vi "Gaussmeter425_BvsTime_HeliumEdition.vi"() -> ()   [LabVIEW 2014]
uses:
  <vilib>/Platform/TimedLoop/XDataNode/timing_clust.ctl
  <vilib>/Platform/TimedLoop/XDataNode/nitl_modes.ctl
  <vilib>/Platform/TimedLoop/XDataNode/wakeup.ctl
  <instrlib>/Agilent 3446X Series/Public/Data/Read (Single Point).vi
  <instrlib>/Lake Shore 425/Public/Data/Field Data (Single Reading).vi
  <vilib>/Utility/file.llb/Write To Spreadsheet File (DBL).vi
  <vilib>/Platform/TimedLoop/XDataNode/XDataNode.xnode
  <instrlib>/Lake Shore 425/Lake Shore 425.lvlib
  <vilib>/Platform/TimedLoop/XDataNode/XDNodeRunTimeDep.lvlib
  <instrlib>/Agilent 3446X Series/Agilent 3446X Series.lvlib
panel:
  out "Output file name":string
  in  "Use multimeter ON / OFF":bool=TRUE
  in  "Comments":string
  in  "Setup":string(combo)
  out "?":dbl(graph)
  in  "VISA resource name MM":refnum<visa-resource-name>="USB0::0x0957::0x1A07::MY53203201::INSTR"
  in  "Measurement Function (10: Voltage DC)":i32(ring)=10 items=["Continuity", "Current AC", "Current DC", "Diode", "Frequency", "Resistance 4-wire", "Period", "Resistance 2-wire", "Temperature", "Voltage AC", "Voltage DC", "Voltage DC Ratio"]
  out "Current [A]":dbl
  out "Magnetic Flux [mT]":dbl
  in  "day":dbl
  in  "h":dbl
  in  "min":dbl
  in  "sec":dbl
  out "Time since run start [s]":dbl
  in  "VISA resource name GM":refnum<visa-resource-name>="COM4"
  in  "Measurements per second:":dbl=1.0
  out "?":dbl(graph)
  in  "?":bool
  in  "Serial Configuration":T1={"Baud Rate"=57600, "Parity"=1, "Data Bits"=7, "Stop Bits"=10, "Flow Control"=0} {"Flow Control" items=["None", "XON/XOFF", "RTS/CTS", "XON/XOFF & RTS/CTS", "DTR/DSR", "XON/XOFF & DTR/DSR"]; "Stop Bits" items=["1.0"=10, "1.5"=15, "2.0"=20]; "Data Bits" items=["7"=7, "8"=8]; "Parity" items=["None", "Odd", "Even", "Mark", "Space"]; "Baud Rate" items=["300"=300, "600"=600, "1200"=1200, "2400"=2400, "4800"=4800, "9600"=9600, "19200"=19200, "38400"=38400, "57600"=57600]}
  # "Automatically stop after..."
  # "more than 3 may not work"
  # "Gaussmeter"
  # "Multimeter"
  # "USB0::0x0957: for multimeter"
  # "Voltage DC for Amp"
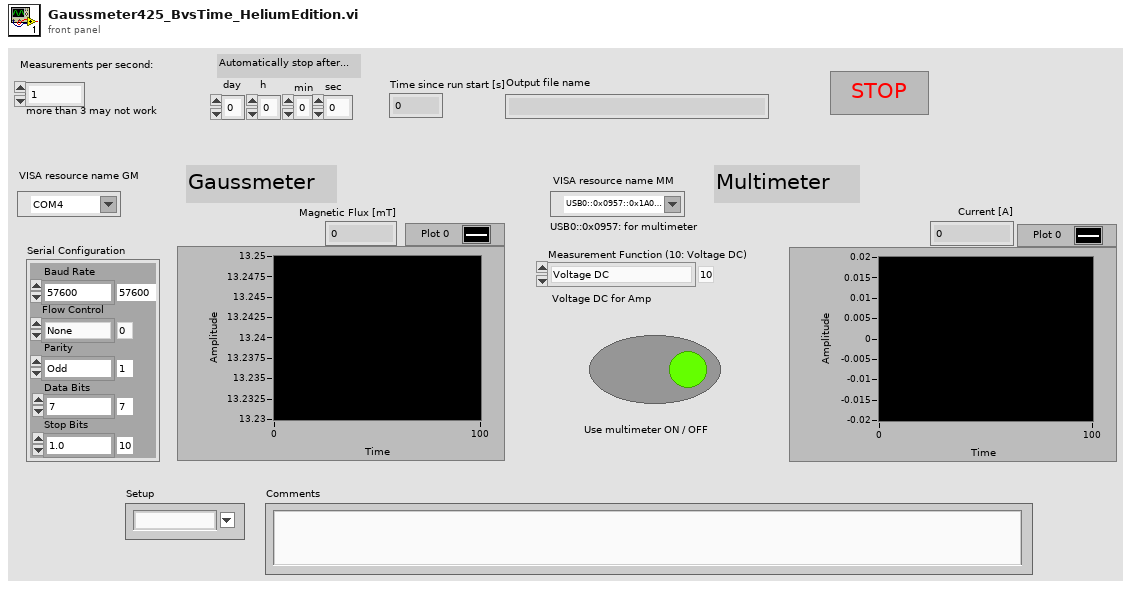
[diagram p1: front panel]
types:
  T1 = cluster{"Baud Rate":u32, "Parity":u16, "Data Bits":u16, "Stop Bits":u16, "Flow Control":u16}
  T2 = typedef "XDNodeRunTimeDep.lvlib/timing_clust.ctl" = cluster{"Expected End [f-1]":u64, "Actual End [f-1]":u64, "Finished Late? [f-1]":bool, "Expected End [i-1]":u64, "Actual End [i-1]":u64, "Finished Late? [i-1]":bool, "Expected Start [i]":u64, "Actual Start [i]":u64, "Expected Start [f]":u64, "Actual Start [f]":u64, "Source Name":string, "Structure Name":string, "Period":i64, "Deadline":i64, "Offset":i64, "Start":i64, "Priority":i32, "Timeout":i32, "Mode":T3, "Wakeup Reason":T4, "Error":errorcluster, "Source Type":string, "Secondary Source Type":string, "Global End Time":u64, "Global Start Time":u64, "Frame Duration":u64, "Iteration Duration":u64, "Assigned CPU":i32, "I/O Scan Engine Mode":u32}
  T3 = typedef "XDNodeRunTimeDep.lvlib/nitl_modes.ctl" = enum32{"No Change", "Process missed periods, maintain original phase", "Discard missed periods, maintain original phase", "Process missed periods, ignore original phase", "Discard missed periods, ignore original phase"}
  T4 = typedef "XDNodeRunTimeDep.lvlib/wakeup.ctl" = enum32{"Normal", "Aborted", "Asynchronous wakeup", "Timing source error", "Timed loop error", "Timeout"}
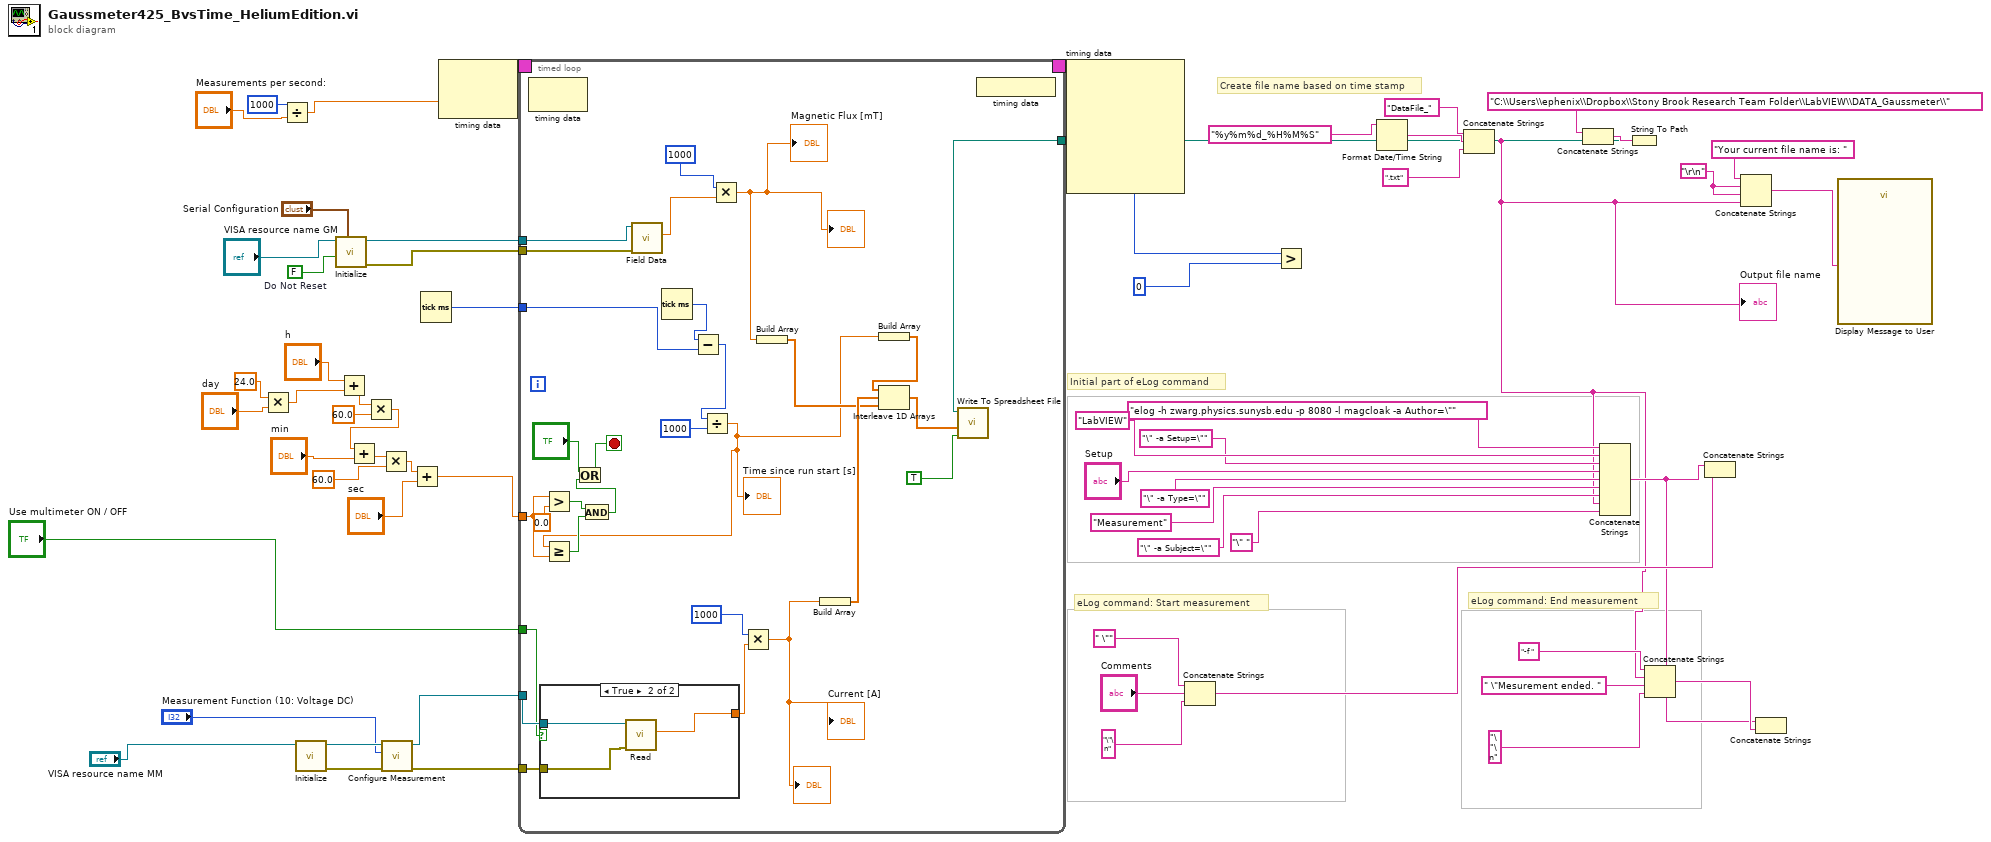
[diagram p0: block diagram]
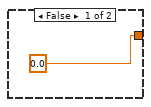
[diagram p2: hidden frame]
diagram:
  w46 = "\r\n"
  w60 = FALSE  # Do Not Reset
  # "eLog command: End measurement"
  # "eLog command: Start measurement"
  # "Initial part of eLog command"
  # "Create file name based on time stamp"
  n1 = Multiply(x=24.0, y="day") -> (x*y=w41:dbl)
  n2 = Divide(x=1000, y="Measurements per second:") -> (x/y=w44:dbl)
  n3 = call <instrlib>:"Initialize.vi"("VISA resource name"="VISA resource name MM") -> ("error out"=w30:errorcluster, "VISA resource name out"=w31:refnum<visa-resource-name>)  [unwired: 4 in, 5 out]
  n4 = call <instrlib>:"Initialize.vi"("Serial Configuration"="Serial Configuration", "Reset (True)"=w60, "VISA resource name"="VISA resource name GM") -> ("error out"=w57:errorcluster, "VISA resource name out"=w58:refnum<visa-resource-name>)  [unwired: 7 in]
  n5 = Add(x="h", y=w41) -> (x+y=w40:dbl)
  n6 = Multiply(x=w40, y=60.0) -> (x*y=w38:dbl)
  n7 = Add(x=w38, y="min") -> (x+y=w36:dbl)
  n8 = Multiply(x=w36, y=60.0) -> (x*y=w34:dbl)
  n9 = call <instrlib>:"Configure Measurement.vi"("error in (no error)"=w30, "Measurement Function (10: Voltage DC)"="Measurement Function (10: Voltage DC)", "VISA resource name"=w31) -> ("error out"=w26:errorcluster, "VISA resource name out"=w27:refnum<visa-resource-name>)  [unwired: 3 in, 4 out]
  n10 = Add(x=w34, y="sec") -> (x+y=w32:dbl)
  n11 = Tick Count (ms)() -> (millisecond timer value=w4:u32)
  n12 = node-c288(w44) -> (w56:T2)  [unwired: 1 in]
  n13 = Concatenate Strings(" \"", "Comments", "\"\n") -> (w12:string)
  n14 = Format Date/Time String(time format string (%c)="%y%m%d_%H%M%S") -> (date/time string=w48:string)  [unwired: 2 in]
  n15 = Concatenate Strings("DataFile_", w48, ".txt") -> (w1:string)
  "Output file name" <- w1
  n16 = Concatenate Strings("C:\\Users\\ephenix\\Dropbox\\Stony Brook Research Team Folder\\LabVIEW\\DATA_Gaussmeter\\", w1) -> (w25:string)
  n17 = Concatenate Strings("elog -h zwarg.physics.sunysb.edu -p 8080 -l magcloak -a Author=\"", "LabVIEW", "\" -a Setup=\"", "Setup", "\" -a Type=\"", "Measurement", "\" -a Subject=\"", w1, "\" ") -> (w5:string)
  n18 = String To Path(string=w25) -> (path=w17:path)
  n19 = timed-loop {
    tunnel: w58 -> [w90]
    tunnel: w57 -> [w89]
    timing: w56 -> [_]
    timing-out: [_] -> w55
    tunnel: w32 -> [w80]
    tunnel: w27 -> [w63]
    tunnel: w26 -> [w64]
    tunnel: w17 -> [w73]
    tunnel: w4 -> [w69]
    tunnel: "Use multimeter ON / OFF" -> [w62]
    stop <- w86 stop-if-true
    n20 = node-c288() -> ()  [unwired: 1 in, 1 out]
    n21 = case shown="True" w62 {
      tunnel: [0.0 w94] -> w78
      tunnel: w64 -> [_ w93]
      tunnel: w63 -> [_ w92]
      frame False {
      }
      frame True {
        n22 = call-poly <instrlib>:"Read.vi"("error in (no error)"=w93, "VISA resource name"=w92) -> ("Measurement"=w94:dbl)  [unwired: 2 in, 7 out]
      }
    }
    n23 = Greater?(x=w80, y=0.0) -> (0:w83:bool)
    n24 = call-poly <instrlib>:"Field Data.vi"("error in (no error)"=w89, "VISA resource name"=w90) -> ("Field Reading"=w87:dbl)  [unwired: 7 in, 2 out]
    n25 = Tick Count (ms)() -> (millisecond timer value=w70:u32)
    n26 = Subtract(x=w70, y=w69) -> (x-y=w68:u32)
    n27 = Divide(x=w68, y=u32 1000) -> (x/y=w65:dbl)
    "Time since run start [s]" <- w65
    n28 = Greater Or Equal?(x=w65, y=w80) -> (x >= y?=w82:bool)
    n29 = And(x=w83, y=w82) -> (x .and. y?=w84:bool)
    n30 = Or(x="?", y=w84) -> (x .or. y?=w86:bool)
    n31 = Multiply(x=1000, y=w87) -> (x*y=w79:dbl)
    "?" <- w79
    "Magnetic Flux [mT]" <- w79
    n32 = Multiply(x=1000, y=w78) -> (x*y=w74:dbl)
    "Current [A]" <- w74
    "?" <- w74
    n33 = Build Array(w79) -> (w75:dbl[])
    n34 = Build Array(w74) -> (w76:dbl[])
    n35 = Build Array(w65) -> (w66:dbl[])
    n36 = Interleave 1D Arrays(w66, w76, w75) -> (w72:dbl[])
    n37 = call-poly <vilib>:"Write To Spreadsheet File.vi"("append to file? (new file:F)"=TRUE, "1D data"=w72, "file path (dialog if empty)"=w73) -> ()  [unwired: 5 in, 1 out]
    n38 = node-c288() -> ()  [unwired: 1 out]
  }
  n39 = node-c288(w55) -> (w10:i64)  [unwired: 6 out]
  n40 = Greater?(x=w10, y=0) -> ()  [unwired: 1 out]
  n41 = Concatenate Strings("-f ", w1, " \"Mesurement ended. ", "\"\n") -> (w8:string)
  n42 = Concatenate Strings(w5, w12) -> ()  [unwired: 1 out]
  n43 = Concatenate Strings("Your current file name is: ", w46, w46, w1) -> (w45:string)
  n44 = Concatenate Strings(w5, w8) -> ()  [unwired: 1 out]
  n45 = call "Display Message to User"("Message"=w45) -> ()  [unwired: 9 in, 2 out]
